vi "IlmaInfoLugeja.vi"() -> ()   [LabVIEW 2020]
uses:
  Downloads/visuaalprogrammeerimine/visuaalprogrammeerimine/Ilmajaamad.ctl
  Downloads/visuaalprogrammeerimine/visuaalprogrammeerimine/Ilmajaam.ctl
  6bc99e37-775f-4bec-abaf-435e326e10ca.vi
  <vilib>/JDP Science/JSONtext/JSON text to Variant.vi
  <vilib>/JDP Science/JSONtext/LVClass Serializer/JSONtext LVClass Serializer.lvclass
panel:
  out "Kõige soojem ilmajaam":string
  out "Array":T1
  in  "file path (use dialog)":path
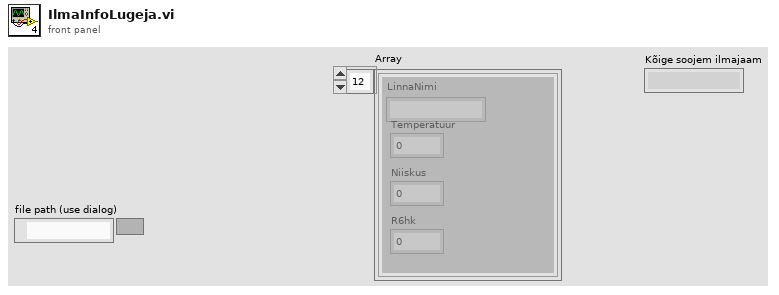
[diagram p1: front panel]
types:
  T1 = typedef "Ilmajaamad.ctl" = T2[]
  T2 = typedef "Ilmajaam.ctl" = cluster{"LinnaNimi":string, "Temperatuur":dbl, "Niiskus":dbl, "R6hk":dbl}
  T3 = cluster{"LinnaNimi":string, "Temperatuur":i32, "Niiskus":i32, "R6hk":i32}[]
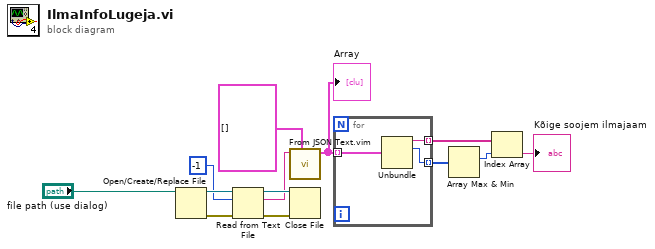
[diagram p0: block diagram]
diagram:
  n1 = Open/Create/Replace File(file path (use dialog)="file path (use dialog)") -> (refnum out=w12:refnum<file>, error out=w13:errorcluster)  [unwired: 5 in, 1 out]
  n2 = Read from Text File(file (use dialog)=w12, count=-1, error in=w13) -> (refnum out=w8:refnum<file>, text=w6:string, error out=w9:errorcluster)  [unwired: 1 in, 1 out]
  n3 = call "From JSON Text.vim"("Data Type and Default Value"=T3 [], "JSON"=w6) -> ("Data out"=w5:T3)  [unwired: 8 in, 1 out]
  "Array" <- w5
  n4 = Close File(refnum=w8, error in=w9) -> ()  [unwired: 2 out]
  n5 = for {
    tunnel: w5 -> [w16] mode=indexing
    tunnel: [w15] -> w4 mode=indexing
    tunnel: [w14] -> w3 mode=indexing
    n6 = Unbundle(w16) -> ("LinnaNimi"=w14:string, "Temperatuur"=w15:i32)  [unwired: 2 out]
  }
  n7 = Array Max & Min(array=w4) -> (max index (indices)=w2:i32)  [unwired: 3 out]
  n8 = Index Array(array=w3, index=w2) -> (element=→"Kõige soojem ilmajaam":string)
